vi "Delacor_lib_QMH_Release Message Queue.vi"(8 "error in":errorcluster, 11 "Message Queue":refnum<class "RQMHMessageQueue.lvclass">) -> (0 "error out":errorcluster)   [LabVIEW 2024, in "RQMHMessageQueue.lvclass"]
doc: "Release the message queue.\n____\nDQMH Framework: Palette 7.1.0.1503\nCopyright (c) 2025, DQMH Consortium"
uses:
  RQMHMessageQueue.lvclass
  RQMHMessageQueue.lvclass/RQMHMessageQueue.ctl
  Delacor_lib_QMH_Get Message Queue.vi
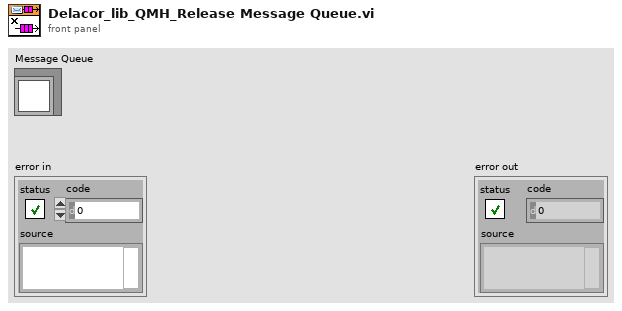
[diagram p1: front panel]
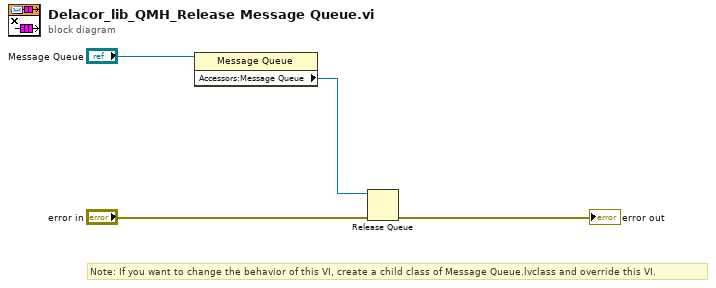
[diagram p0: block diagram]
diagram:
  # "Note: If you want to change the behavior of this VI, create a child class of Message Queue.lvclass and override this VI."
  n1 = property class="Message Queue"(reference="Message Queue") -> ("Accessors:Message Queue"=w1:refnum<queue>)  [unwired: 1 in, 2 out]
  n2 = Release Queue(queue=w1, error in (no error)="error in") -> (error out=→"error out":errorcluster)  [unwired: 1 in, 2 out]
